vi "Get Session Manager Client.vi"(8 "error in (no error)":errorcluster, 11 "ClientPool in":refnum<class "ClientPool.lvclass">) -> (0 "error out":errorcluster, 2 "Session manger grpc id":T1, 3 "ClientPool out":refnum<class "ClientPool.lvclass">)   [LabVIEW 2020, in "MeasurementLink Measurement Server.lvlib" / "ClientPool.lvclass"]
uses:
  ClientPool.lvclass
  <vilib>/gRPC/LabVIEW gRPC Library/Shared/grpcId.ctl
  ClientPool.lvclass/ClientPool.ctl
  MeasurementLink Discovery Client/RPC Messages/ni_measurementlink_discovery_v1_ResolveServiceRequest.ctl
  MeasurementLink Discovery Client/MeasurementLink Discovery Client.lvlib
  MeasurementLink Session Management Client/MeasurementLink Session Management Client.lvlib
  MeasurementLink Measurement Server.lvlib
  <vilib>/gRPC/LabVIEW gRPC Library/grpc-lvsupport-release.lvlib
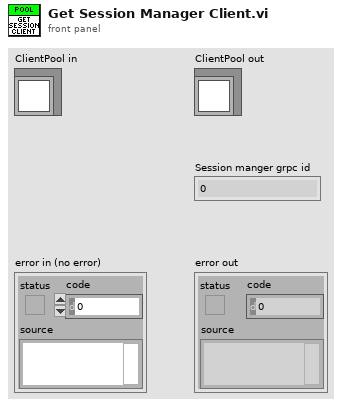
[diagram p1: front panel]
types:
  T1 = typedef "grpc-lvsupport-release.lvlib/grpcId.ctl" = u64
  T2 = typedef "MeasurementLink Discovery Client.lvlib/ni_measurementlink_discovery_v1_ResolveServiceRequest.ctl" = cluster{"provided_interface":string, "service_class":string}
  T3 = typedef "MeasurementLink Discovery Client.lvlib/ni_measurementlink_discovery_v1_ServiceLocation.ctl" = cluster{"location":string, "insecure_port":string, "ssl_authenticated_port":string}
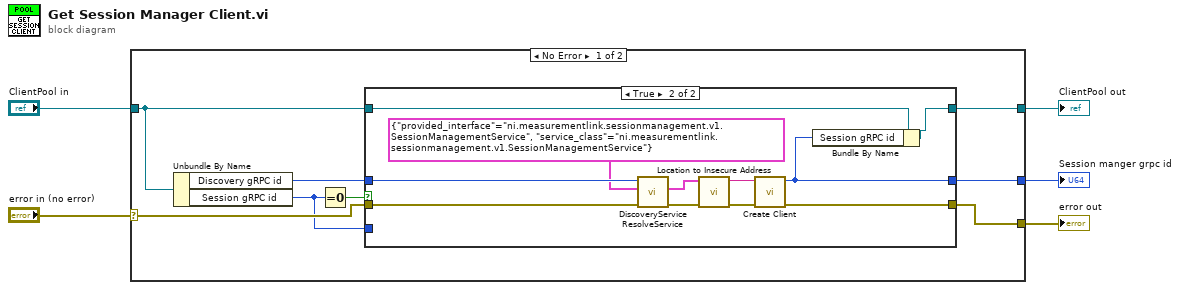
[diagram p0: block diagram]
diagram:
  n1 = case shown="No Error" "error in (no error)" {
    selector: "error in (no error)" -> [w11 w28]
    tunnel: [w10 w28] -> w4
    tunnel: [w6 w27] -> w2
    tunnel: "ClientPool in" -> [w7 w27]
    tunnel: [w8 _] -> w1
    frame No Error {
      n2 = Unbundle By Name(w7) -> ("Discovery gRPC id"=w12:T1, "Session gRPC id"=w9:T1)
      n3 = Equal To 0?(x=w9) -> (x = 0?=w13:bool)
      n4 = case shown="True" w13 {
        tunnel: w12 -> [_ w25]
        tunnel: w11 -> [w16 w24]
        tunnel: [w15 w19] -> w8
        tunnel: [w16 w23] -> w10
        tunnel: w9 -> [w15 _]
        tunnel: w7 -> [w14 w21]
        tunnel: [w14 w20] -> w6
        frame False {
        }
        frame True {
          n5 = call "DiscoveryService ResolveService.vi"("error in"=w24, "Request Data"=T2 {"provided_interface"="ni.measurementlink.sessionmanagement.v1.SessionManagementService", "service_class"="ni.measurementlink.sessionmanagement.v1.SessionManagementService"}, "gRPC ID"=w25) -> ("error out"=w26:errorcluster, "Response Data"=w18:T3)  [unwired: 6 in, 1 out]
          n6 = call "Location to Insecure Address.vi"("Location"=w18) -> ("Address"=w17:string)  [unwired: 10 in]
          n7 = call "Create Client.vi"("error in"=w26, "address"=w17) -> ("error out"=w23:errorcluster, "gRPC ID Out"=w19:T1)  [unwired: 8 in]
          n8 = Bundle By Name(cluster=w21, "Session gRPC id"=w19) -> (w20:refnum<class "ClientPool.lvclass">)
        }
      }
    }
    frame Error {
    }
  }
  "error out" <- w4
  "ClientPool out" <- w2
  "Session manger grpc id" <- w1
